vi "Set Plugin Settings UI.vi"(8 "error in (no error)":errorcluster, 10 "Plugin Settings UI":refnum<class "User Interface.lvclass">, 11 "Component UI in":refnum<class "Component User Interface.lvclass">) -> (0 "error out":errorcluster, 3 "Component UI out":refnum<class "Component User Interface.lvclass">)   [LabVIEW 2017, in "DSF Core.lvlib" / "Component User Interface.lvclass"]
uses:
  Component User Interface.lvclass
  User Interface/User Interface.lvclass
  Component User Interface.lvclass/Component User Interface.ctl
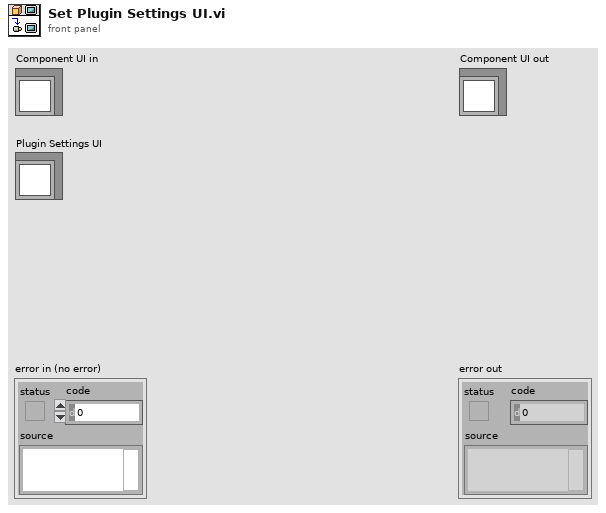
[diagram p1: front panel]
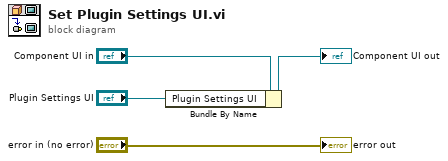
[diagram p0: block diagram]
diagram:
  n1 = Bundle By Name(cluster="Component UI in", "Plugin Settings UI"="Plugin Settings UI") -> (→"Component UI out":refnum<class "Component User Interface.lvclass">)
  "error out" <- "error in (no error)"
